vi "Cambiar contraseña.vi"(8 "error in":errorcluster) -> (0 "error out":errorcluster)   [LabVIEW 2017]
uses:
  Globals/Global.vi
panel:
  in  "Cancel":bool
  in  "OK":bool
  in  "Confirmar nueva contraseña":string
  in  "Nueva contraseña":string
  in  "Contraseña actual":string
  in  "Usuario":string
  # "CAMBIAR CONTRASEÑA"
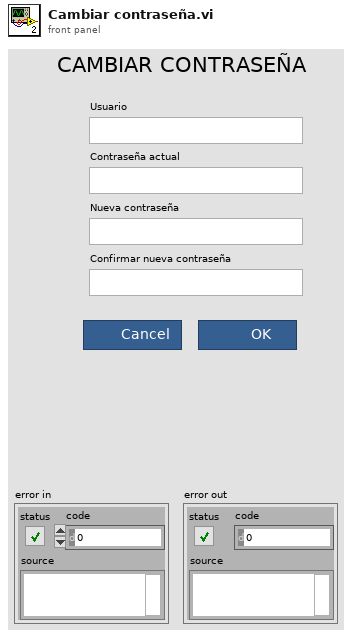
[diagram p1: front panel]
types:
  T1 = cluster{"Nombre de usuario":string, "Contraseña":string, "Trabajador":string}[]
  T2 = cluster{"Nombre de usuario":string, "Contraseña":string, "Trabajador":string}
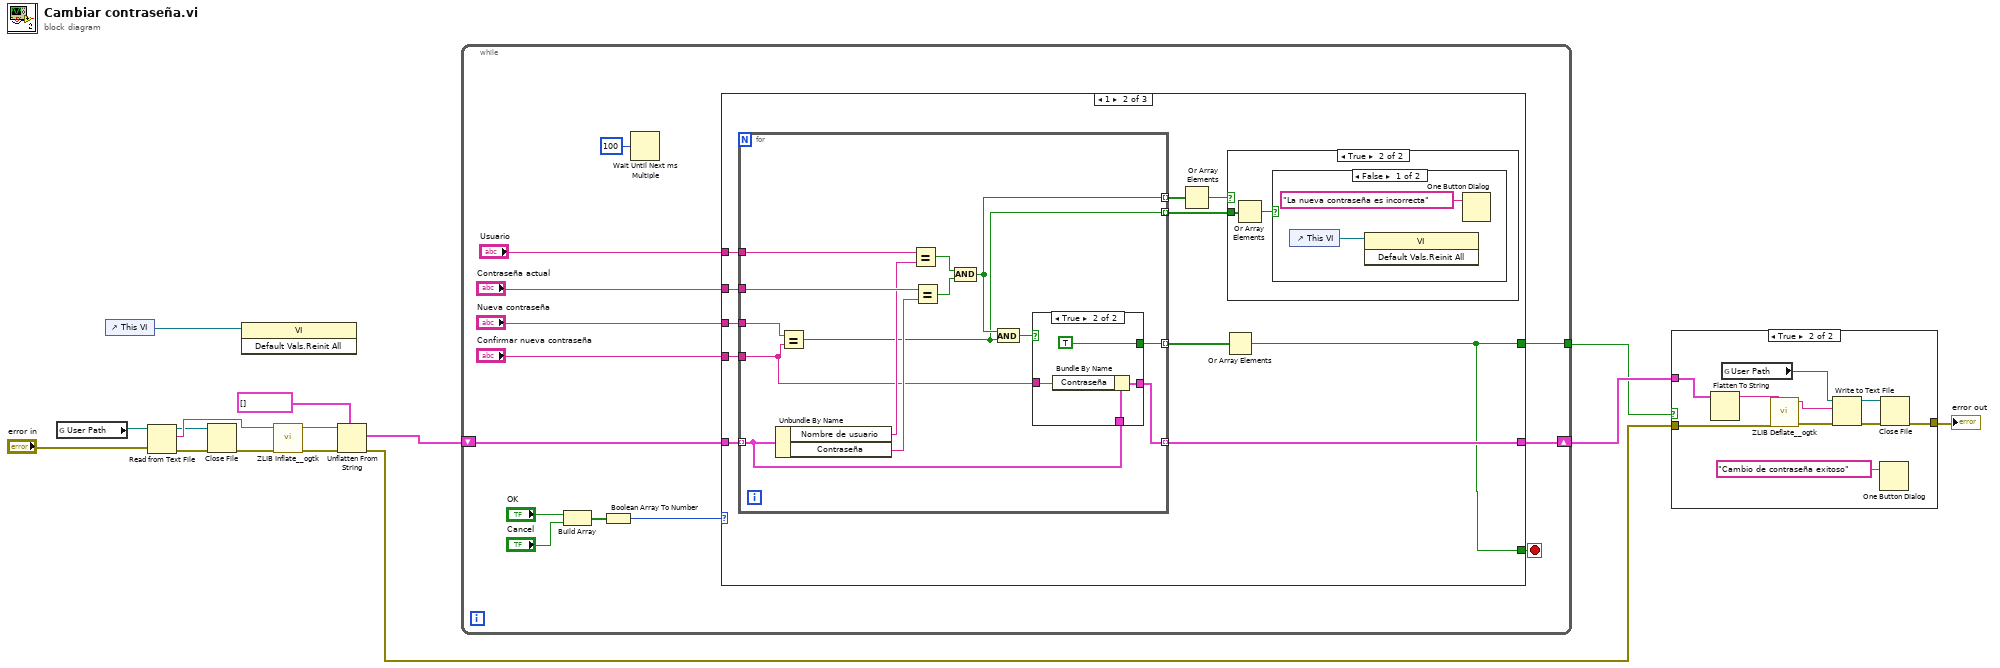
[diagram p0: block diagram]
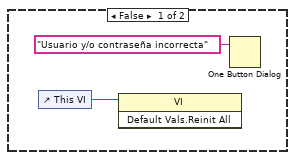
[diagram p3: hidden frame]
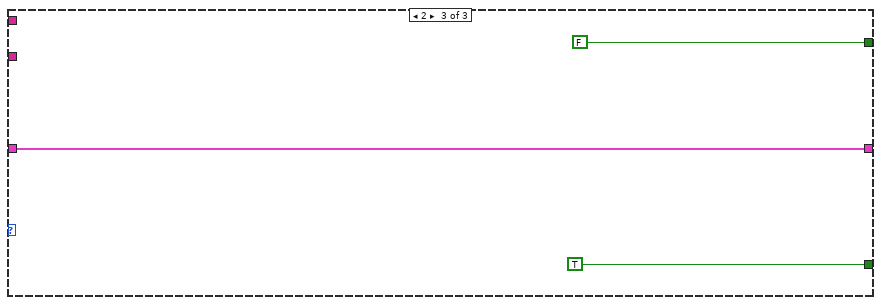
[diagram p6: hidden frame]
diagram:
  n1 = global read "Global.vi" "User Path"() -> (w12:path)
  n2 = control-ref of="This VI"() -> (w6:refnum<vi>)
  n3 = Read from Text File(file (use dialog)=w12, error in="error in") -> (refnum out=w3:refnum<file>, text=w13:string, error out=w2:errorcluster)  [unwired: 2 in, 1 out]
  n4 = Close File(refnum=w3, error in=w2) -> (error out=w1:errorcluster)  [unwired: 1 out]
  n5 = invoke class="VI" method="Default Vals.Reinit All"(reference=w6) -> ()  [unwired: 2 in, 3 out]
  n6 = call <userlib>:"ZLIB Inflate__ogtk.vi"("error in (no error)"=w1, "input"=w13) -> ("error out"=w14:errorcluster, "inflated output"=w4:string)  [unwired: 3 in, 1 out]
  n7 = Unflatten From String(type=T1 [] ("Array"), binary string=w4, error in (no error)=w14) -> (value=w11:T1, error out=w9:errorcluster)  [unwired: 2 in, 1 out]
  n8 = while {
    shift-right: [w23] -> w10
    shift-left: w11 -> [w28]
    tunnel: [w22] -> w8
    stop <- w17 stop-if-true
    n9 = Build Array("OK", "Cancel") -> (w19:bool[])
    n10 = Boolean Array To Number(Boolean array=w19) -> (number=w18:u32)
    n11 = Wait Until Next ms Multiple(millisecond multiple=u32 100) -> ()  [unwired: 1 out]
    n12 = case shown="1" w18 {
      tunnel: w28 -> [w29 w40 w66]
      tunnel: "Usuario" -> [_ w39 _]
      tunnel: "Contraseña actual" -> [_ w38 _]
      tunnel: "Nueva contraseña" -> [_ w37 _]
      tunnel: "Confirmar nueva contraseña" -> [_ w36 _]
      tunnel: [w29 w35 w66] -> w23
      tunnel: [_ w33 FALSE] -> w22
      tunnel: [_ w33 TRUE] -> w17
      frame 0, Default {
      }
      frame 1 {
        n13 = for {
          tunnel: w40 -> [w53] mode=indexing
          tunnel: w39 -> [w60]
          tunnel: w38 -> [w59]
          tunnel: w37 -> [w54]
          tunnel: w36 -> [w52]
          tunnel: [w51] -> w35 mode=indexing
          tunnel: [w49] -> w34 mode=indexing
          tunnel: [w48] -> w32 mode=indexing
          tunnel: [w47] -> w30 mode=indexing
          n14 = Unbundle By Name(w53) -> ("Nombre de usuario"=w57:string, "Contraseña"=w58:string)
          n15 = Equal?(x=w54, y=w52) -> (x = y?=w47:bool)
          n16 = Equal?(x=w60, y=w57) -> (x = y?=w56:bool)
          n17 = Equal?(x=w59, y=w58) -> (x = y?=w55:bool)
          n18 = And(x=w56, y=w55) -> (x .and. y?=w48:bool)
          n19 = And(x=w48, y=w47) -> (x .and. y?=w50:bool)
          n20 = case shown="True" w50 {
            tunnel: w53 -> [w61 w65]
            tunnel: w52 -> [_ w64]
            tunnel: [w61 w63] -> w51
            tunnel: [_ TRUE] -> w49
            frame False {
            }
            frame True {
              n21 = Bundle By Name(cluster=w65, "Contraseña"=w64) -> (w63:T2)
            }
          }
        }
        n22 = Or Array Elements(Boolean array=w32) -> (logical OR=w31:bool)
        n23 = Or Array Elements(Boolean array=w34) -> (logical OR=w33:bool)
        n24 = case shown="True" w31 {
          tunnel: w30 -> [_ w44]
          frame False {
            n25 = control-ref of="This VI"() -> (w41:refnum<vi>)
            n26 = invoke class="VI" method="Default Vals.Reinit All"(reference=w41) -> ()  [unwired: 2 in, 3 out]
            n27 = One Button Dialog(message="Usuario y/o contraseña incorrecta") -> ()  [unwired: 1 in, 1 out]
          }
          frame True {
            n28 = Or Array Elements(Boolean array=w44) -> (logical OR=w43:bool)
            n29 = case shown="False" w43 {
              frame False {
                n30 = control-ref of="This VI"() -> (w45:refnum<vi>)
                n31 = invoke class="VI" method="Default Vals.Reinit All"(reference=w45) -> ()  [unwired: 2 in, 3 out]
                n32 = One Button Dialog(message="La nueva contraseña es incorrecta") -> ()  [unwired: 1 in, 1 out]
              }
              frame True {
              }
            }
          }
        }
      }
      frame 2 {
      }
    }
  }
  n33 = case shown="True" w8 {
    tunnel: w10 -> [_ w73]
    tunnel: w9 -> [w69 w75]
    tunnel: [w69 w70] -> w7
    frame False {
    }
    frame True {
      n34 = Flatten To String(anything=w73) -> (data string=w77:string)  [unwired: 3 in, 2 out]
      n35 = global read "Global.vi" "User Path"() -> (w76:path)
      n36 = call <userlib>:"ZLIB Deflate__ogtk.vi"("error in (no error)"=w75, "input"=w77) -> ("error out"=w78:errorcluster, "deflated output"=w79:string)  [unwired: 3 in, 1 out]
      n37 = Write to Text File(file (use dialog)=w76, text=w79, error in=w78) -> (refnum out=w72:refnum<file>, error out=w71:errorcluster)  [unwired: 1 in, 1 out]
      n38 = One Button Dialog(message="Cambio de contraseña exitoso") -> ()  [unwired: 1 in, 1 out]
      n39 = Close File(refnum=w72, error in=w71) -> (error out=w70:errorcluster)  [unwired: 1 out]
    }
  }
  "error out" <- w7
